vi "Handle Server Request.vi"(8 "error in (no error)":errorcluster, 9 "Data":string, 10 "Method":string, 11 "Sequencer in":refnum<class "Sequencer.lvclass">) -> (0 "error out":errorcluster, 2 "Response":string, 3 "Sequencer out":refnum<class "Sequencer.lvclass">)   [LabVIEW 2024, in "Ramses Sequencer.lvlib" / "Sequencer.lvclass"]
uses:
  Sequencer.lvclass
  Program Files (x86)/Enterative/Ramses Framework/Ramses Framework.lvlibp/Service/Service.lvclass
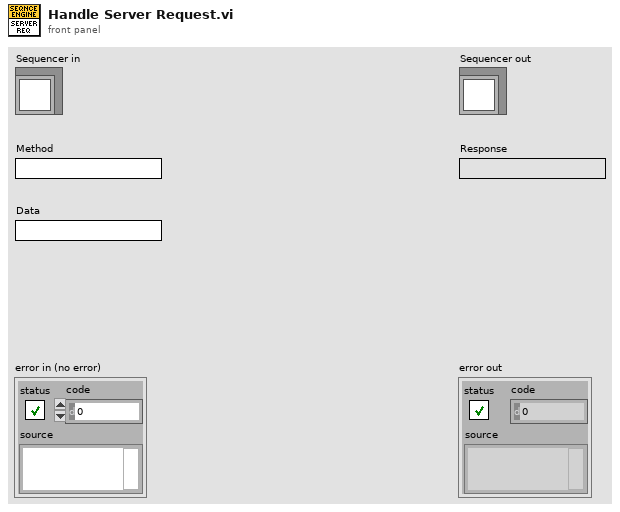
[diagram p1: front panel]
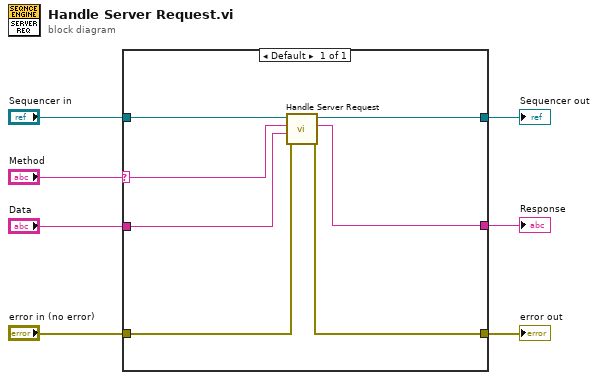
[diagram p0: block diagram]
diagram:
  n1 = case shown="Default" "Method" {
    selector: "Method" -> [w12]
    tunnel: "Sequencer in" -> [w14]
    tunnel: "Data" -> [w13]
    tunnel: "error in (no error)" -> [w11]
    tunnel: [w10] -> w3
    tunnel: [w9] -> w4
    tunnel: [w8] -> w5
    frame Default {
      n2 = call-parent "Handle Server Request.vi"("error in (no error)"=w11, "Data"=w13, "Method"=w12, "Service in"=w14) -> ("error out"=w10:errorcluster, "Response"=w9:string, "Service out"=w8:refnum<class "Sequencer.lvclass">)  [unwired: 5 in]
    }
  }
  "error out" <- w3
  "Sequencer out" <- w5
  "Response" <- w4
